vi "Helper - Camera Identification.vi"() -> ()   [LabVIEW 2011]
uses:
  <vilib>/vision/driver/NI_Vision_Acquisition_Software.lvlib
panel:
  out "Image":T1(plugin-control)
  out "Camera Info":T2 {"SerialNumberHigh" format="%x"; "SerialNumberLow" format="%x"}
  out "error out":errorcluster
  in  "Get Image":bool
  in  "camera number":i32
  in  "stop":bool
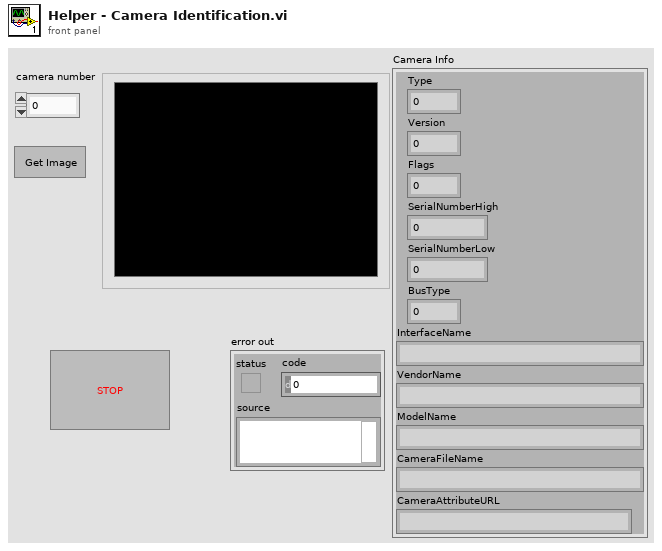
[diagram p1: front panel]
types:
  T1 = typedef "IMAQ Image.ctl" = refnum<image>
  T2 = cluster{"Type":u32, "Version":u32, "Flags":u32, "SerialNumberHigh":u32, "SerialNumberLow":u32, "BusType":u32, "InterfaceName":string, "VendorName":string, "ModelName":string, "CameraFileName":string, "CameraAttributeURL":string}
  T3 = cluster{"Type":u32, "Version":u32, "Flags":u32, "SerialNumberHigh":u32, "SerialNumberLow":u32, "BusType":u32, "InterfaceName":string, "VendorName":string, "ModelName":string, "CameraFileName":string, "CameraAttributeURL":string}[]
  T4 = typedef "IMAQdx.ctl" = refnum<k21>
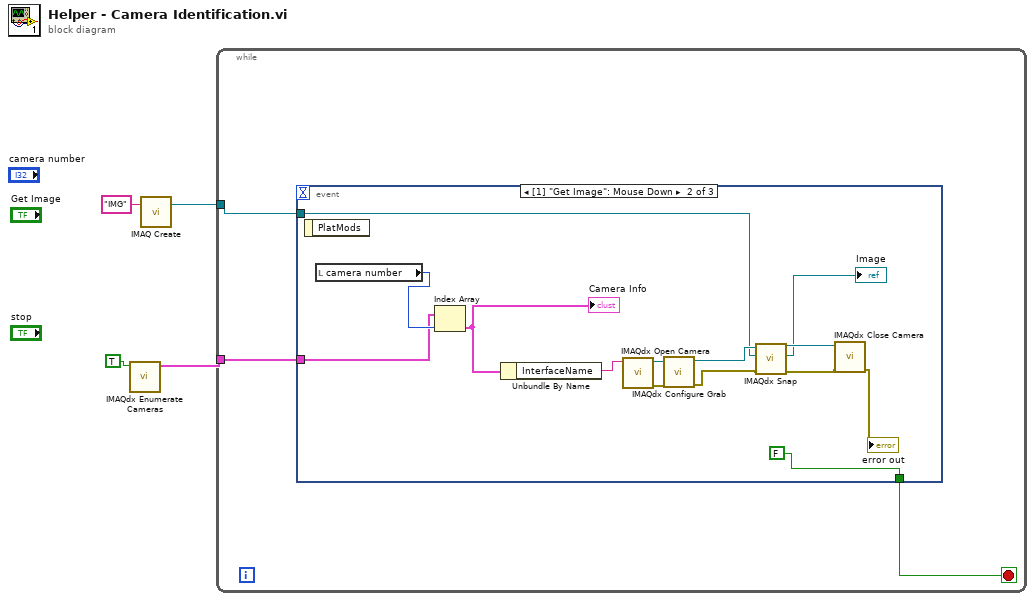
[diagram p0: block diagram]
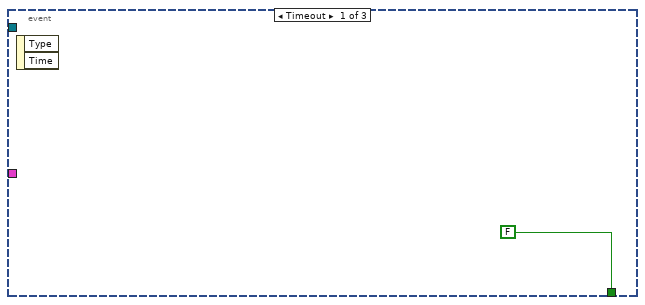
[diagram p2: hidden frame]
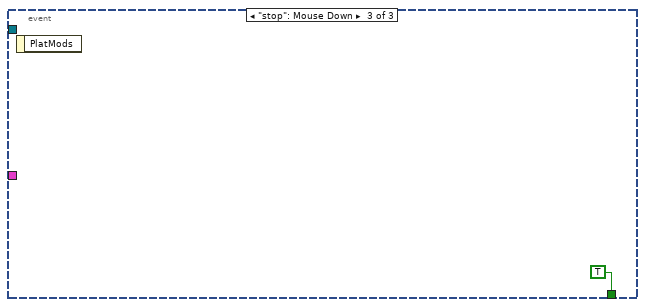
[diagram p3: hidden frame]
diagram:
  n1 = call <vilib>:"IMAQdx Enumerate Cameras.vi"("Connected Only? (Yes)"=TRUE) -> ("Camera Information Array"=w1:T3)  [unwired: 9 in, 1 out]
  n2 = call "IMAQ Create"("Image Name"="IMG") -> ("New Image"=w3:T1)  [unwired: 4 in, 1 out]
  n3 = while {
    tunnel: w3 -> [w7]
    tunnel: w1 -> [w6]
    stop <- w5 stop-if-true
    n4 = event shown="[1] \"Get Image\": Mouse Down" {
      selector: _ -> [_ _ _]
      dyn-events: _ -> [_ _ _]
      timeout: _ -> [_ _ _]
      tunnel: w7 -> [_ w10 _]
      tunnel: w6 -> [_ w12 _]
      tunnel: [FALSE FALSE TRUE] -> w5
      event Timeout {
        n5 = event-data() -> ()  [unwired: 1 in, 2 out]
      }
      event "Get Image": Mouse Down {
        n6 = event-data() -> ()  [unwired: 1 in, 1 out]
        n7 = local read "camera number"() -> (w22:i32)
        n8 = Index Array(array=w12, index=w22) -> (element=w16:T2)
        "Camera Info" <- w16
        n9 = Unbundle By Name(w16) -> ("InterfaceName"=w13:string)
        n10 = call <vilib>:"IMAQdx Open Camera.vi"("Session In"=w13) -> ("error out"=w15:errorcluster, "Session Out"=w14:T4)  [unwired: 9 in]
        n11 = call <vilib>:"IMAQdx Configure Grab.vi"("error in"=w15, "Session In"=w14) -> ("error out"=w18:errorcluster, "Session Out"=w17:T4)  [unwired: 8 in]
        n12 = call <vilib>:"IMAQdx Snap.vi"("error in"=w18, "Image In"=w10, "Session In"=w17) -> ("error out"=w21:errorcluster, "Image Out"=→"Image":T1, "Session Out"=w20:T4)  [unwired: 6 in]
        n13 = call <vilib>:"IMAQdx Close Camera.vi"("error in"=w21, "Session In"=w20) -> ("error out"=→"error out":errorcluster)  [unwired: 9 in]
      }
      event "stop": Mouse Down {
        n14 = event-data() -> ()  [unwired: 1 in, 1 out]
      }
    }
  }
